vi "PCC Relay.vi"(8 "error in (no error)":errorcluster, 10 "Relay Name":string, 11 "SCADA in":refnum<class "SCADA.lvclass">) -> (0 "error out":errorcluster, 3 "SCADA out":refnum<class "SCADA.lvclass">)   [LabVIEW 2015, in "SCADA Core.lvlib" / "SCADA.lvclass"]
uses:
  SCADA.lvclass
  Controls/Queue Selector.ctl
  <vilib>/Utility/error.llb/DialogType.ctl
  SCADA Abstract Messages/Device Action Status Msg/Device Action Status.ctl
  SCADA.lvclass/SCADA.ctl
  <vilib>/ActorFramework/Actor/Actor.lvclass/Actor.ctl
  <vilib>/ActorFramework/Actor/Actor.lvclass
  SCADA Abstract Messages/Device Action Status Msg/Device Action Status Msg.lvclass
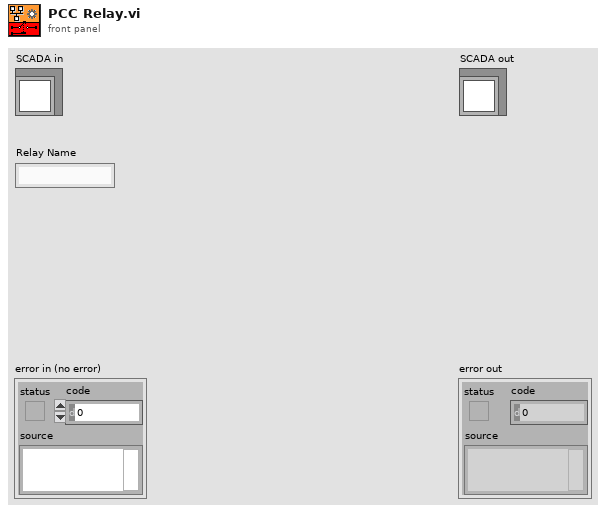
[diagram p1: front panel]
types:
  T1 = typedef "SCADA Core.lvlib/SCADA.lvclass/Queue Selector.ctl" = enum16{"IEDs", "PV", "Generators", "Wind", "Storage", "Relays"}
  T2 = typedef "SCADA Core.lvlib/Device Action Status Msg.lvclass/Device Action Status.ctl" = enum16{"Success", "Failure"}
  T3 = typedef "DialogType.ctl" = u16
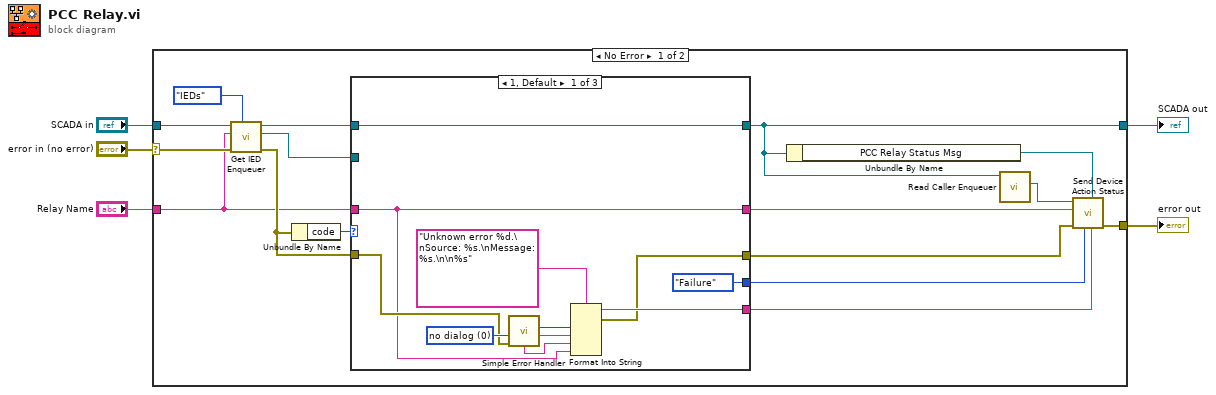
[diagram p0: block diagram]
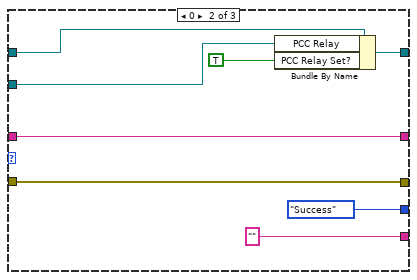
[diagram p2: hidden frame]
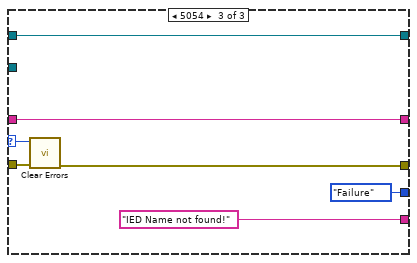
[diagram p3: hidden frame]
diagram:
  n1 = case shown="No Error" "error in (no error)" {
    selector: "error in (no error)" -> [w19 w49]
    tunnel: [w8 w49] -> w2
    tunnel: [w13 w48] -> w1
    tunnel: "SCADA in" -> [w20 w48]
    tunnel: "Relay Name" -> [w16 _]
    frame No Error {
      n2 = call "Get IED Enqueuer.vi"("Queue (IEDs)"=Queue_Selector."IEDs" ("Queue"), "error in (no error)"=w19, "IED Name"=w16, "SCADA in"=w20) -> ("error out"=w17:errorcluster, "IED Enqueuer"=w14:refnum<class "Message Enqueuer.lvclass">, "SCADA out"=w15:refnum<class "SCADA.lvclass">)  [unwired: 5 in]
      n3 = Unbundle By Name(w17) -> ("code"=w18:i32)
      n4 = case shown="1, Default" w18 {
        selector: w18 -> [_ _ w46]
        tunnel: w17 -> [w27 w40 w47]
        tunnel: [w25 w40 w45] -> w9
        tunnel: [w26 "" ("error string") "IED Name not found!" ("error string")] -> w7
        tunnel: [w24 w38 w42] -> w10
        tunnel: w16 -> [w24 w38 w42]
        tunnel: w15 -> [w23 w37 w43]
        tunnel: w14 -> [_ w36 _]
        tunnel: [w23 w35 w43] -> w13
        tunnel: [Device_Action_Status."Failure" ("Status") Device_Action_Status."Success" ("Status") Device_Action_Status."Failure" ("Status")] -> w6
        frame 1, Default {
          w28 = T3 0 items=["no dialog", "OK message", "continue or stop message", "OK message + warnings", "continue/stop + warnings"] ("type of dialog (OK msg:1)")
          n5 = call <vilib>:"Simple Error Handler.vi"("type of dialog (OK msg:1)"=w28, "error in (no error)"=w27) -> ("code out"=w30:i32, "source out"=w31:string, "message"=w32:string)  [unwired: 3 in, 2 out]
          n6 = Format Into String(format string="Unknown error %d.\nSource: %s.\nMessage: %s.\n\n%s" ("Error String"), w30, w31, w32, w24) -> (resulting string=w26:string, error out=w25:errorcluster)  [unwired: 2 in]
        }
        frame 0 {
          n7 = Bundle By Name(cluster=w37, "PCC Relay"=w36, "PCC Relay Set?"=TRUE ("Frequency Control Set?")) -> (w35:refnum<class "SCADA.lvclass">)
        }
        frame 5054 {
          n8 = call <vilib>:"Clear Errors.vi"("error in (no error)"=w47, "specific error code to clear (0: all)"=w46) -> ("error out"=w45:errorcluster)  [unwired: 4 in, 1 out]
        }
      }
      n9 = Unbundle By Name(w13) -> ("PCC Relay Status Msg"=w11:refnum<class "Device Action Status Msg.lvclass">)
      n10 = call <vilib>:"Read Caller Enqueuer.vi"("Actor"=w13) -> ("Caller Enqueuer"=w12:refnum<class "Message Enqueuer.lvclass">)  [unwired: 10 in]
      n11 = call "Send Device Action Status.vi"("error string"=w7, "Island Control Status Msg"=w11, "Status"=w6, "error in (no error)"=w9, "IED Name"=w10, "Message Enqueuer in"=w12) -> ("error out"=w8:errorcluster)  [unwired: 4 in, 1 out]
    }
    frame Error {
    }
  }
  "error out" <- w2
  "SCADA out" <- w1
